vi "Status Created.vi"(7 "jettl in":refnum<class "jettl.lvclass">, 10 "Addresses DVR":refnum<data-value>) -> (0 "Created Count":i32, 1 "Created Aliases":string[](array[string]), 2 "Created Exist?":bool, 5 "jettl out":refnum<class "jettl.lvclass">)   [LabVIEW 2021, in "jettl.lvlib" / "Addresses.lvlib"]
uses:
  Addresses.lvlib
  Addresses/Addresses.lvclass
  jettl/jettl.lvclass
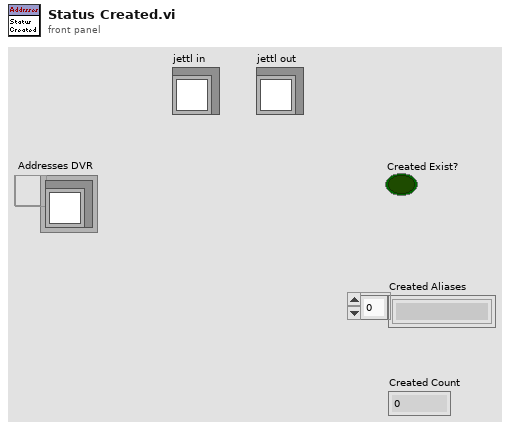
[diagram p1: front panel]
types:
  T1 = typedef "jettl.lvlib/Addresses.lvlib/Created.ctl" = map{string, refnum<class "Msg Type Strategy.lvclass">}
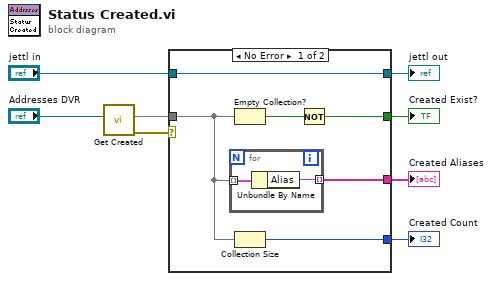
[diagram p0: block diagram]
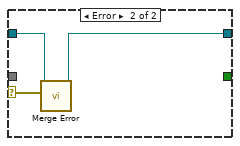
[diagram p2: hidden frame]
diagram:
  n1 = call "Get Created.vi"("Addresses DVR"="Addresses DVR") -> ("error out"=w1:errorcluster, "Created"=w4:T1)  [unwired: 9 in]
  n2 = case shown="No Error" w1 {
    selector: w1 -> [_ w17]
    tunnel: [w13 _] -> w8
    tunnel: [w12 _] -> w7
    tunnel: [w11 _] -> w6
    tunnel: w4 -> [w10 _]
    tunnel: [w9 w18] -> w3
    tunnel: "jettl in" -> [w9 w19]
    frame No Error {
      n3 = for {
        tunnel: [w15] -> w12 mode=indexing
        tunnel: w10 -> [w16] mode=indexing
        n4 = Unbundle By Name(w16) -> ("Alias"=w15:string)
      }
      n5 = Empty Collection?(1:w10) -> (0:w14:bool)
      n6 = Collection Size(1:w10) -> (0:w11:i32)
      n7 = Not(x=w14) -> (.not. x?=w13:bool)
    }
    frame Error {
      n8 = call-dynamic "Merge Error.vi"("Error"=w17, "Merge Error in"=w19) -> ("Merge Error out"=w18:refnum<class "jettl.lvclass">)  [unwired: 9 in]
    }
  }
  "Created Aliases" <- w7
  "Created Exist?" <- w8
  "Created Count" <- w6
  "jettl out" <- w3
